vi "FGV Status LB.vi"(10 "Status in":T1, 11 "command":enum16{"set", "get", "reset"}(ring)=enum."get") -> (2 "Status out":T1)   [LabVIEW 2011]
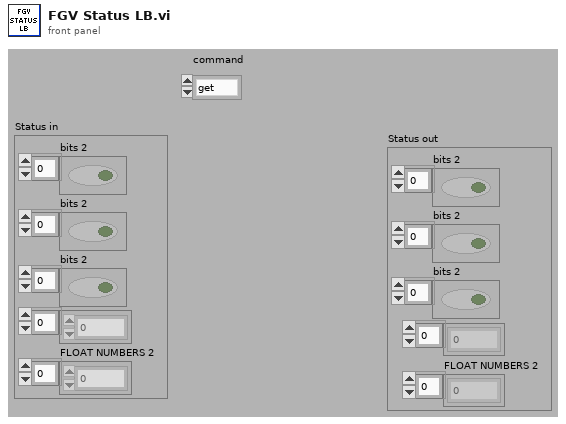
[diagram p1: front panel]
types:
  T1 = cluster{"bits 2":bool[], "bits 2":bool[], "bits 2":bool[], i32[], "FLOAT NUMBERS 2":sgl[]}
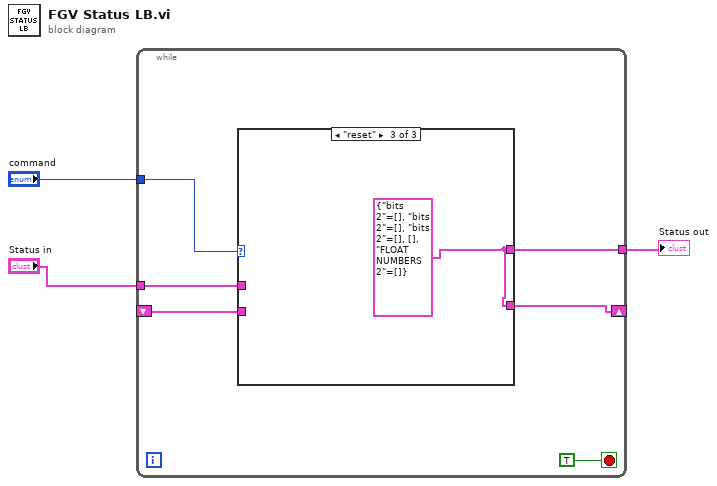
[diagram p0: block diagram]
diagram:
  n1 = while {
    shift-right: [w5] -> _
    shift-left: _ -> [w7]
    tunnel: "command" -> [w8]
    tunnel: [w6] -> w2
    tunnel: "Status in" -> [w4]
    stop <- TRUE stop-if-true
    n2 = case shown="\"reset\"" w8 {
      tunnel: [w10 w11 w12] -> w6
      tunnel: w7 -> [_ w11 _]
      tunnel: [w10 w11 w12] -> w5
      tunnel: w4 -> [w10 _ _]
      frame "set" {
      }
      frame "get", Default {
      }
      frame "reset" {
        w12 = T1 {"bits 2"=[], "bits 2"=[], "bits 2"=[], [], "FLOAT NUMBERS 2"=[]} ("Status 2")
      }
    }
  }
  "Status out" <- w2
